vi "getSquareCoordinates.vi"(10 "Grid":T2, 11 "square":T1) -> (3 "Cluster":cluster{dbl, dbl, dbl, dbl})   [LabVIEW 2020]
uses:
  <vilib>/imath/engines/lvmath2/RunTimeEngine/NodeEndStatement/NIMS_NodeEndStatement_Output.vi
  <instcachedir>/0/NIMS_NodeEndStatement_Output_53EC0D466D134D7ABD903AC30B43404B.lvgen/NIMS_NodeEndStatement_Output_53EC0D466D134D7ABD903AC30B43404B_000.vi
  <vilib>/imath/engines/lvmath2/RunTimeEngine/ErrorHandling/NIMS_Finalize Error.vi
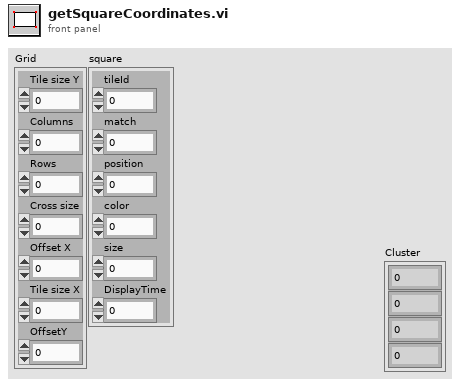
[diagram p1: front panel]
types:
  T1 = cluster{"tileId":i32, "match":i32, "position":i32, "color":u32, "size":i32, "DisplayTime":i32}
  T2 = cluster{"Tile size Y":dbl, "Columns":dbl, "Rows":dbl, "Cross size":dbl, "Offset X":dbl, "Tile size X":dbl, "OffsetY":dbl}
  T3 = cluster{"left":dbl, "top":dbl, "right":dbl, "bottom":dbl}
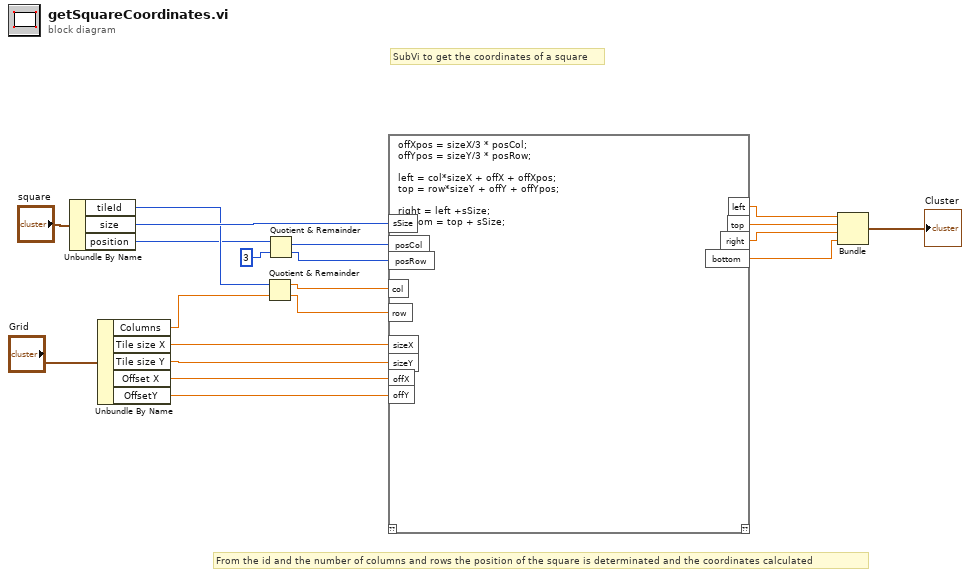
[diagram p0: block diagram]
diagram:
  # "From the id and the number of columns and rows the position of the square is determinated and the coordinates calculated"
  # "SubVi to get the coordinates of a square"
  n1 = Unbundle By Name("square") -> ("tileId"=w17:i32, "size"=w18:i32, "position"=w5:i32)
  n2 = Unbundle By Name("Grid") -> ("Columns"=w16:dbl, "Tile size X"=w13:dbl, "Tile size Y"=w12:dbl, "Offset X"=w11:dbl, "OffsetY"=w10:dbl)
  n3 = Quotient & Remainder(x=w17, y=w16) -> (x-y*floor(x/y)=w15:dbl, floor(x/y)=w14:dbl)
  n4 = Quotient & Remainder(x=w5, y=3) -> (x-y*floor(x/y)=w3:i32, floor(x/y)=w2:i32)
  n5 = mathscript code="offXpos = sizeX/3 * posCol;\noffYpos = sizeY/3 * posRow;\n\nleft = col*sizeX + offX + offXpos;\ntop = row*sizeY + offY + offYpos;\n\nright = left +sSize;\nbottom = top + sSize;"("col"=w15, "row"=w14, "sizeX"=w13, "sizeY"=w12, "sSize"=w18, "offX"=w11, "offY"=w10, "posCol"=w3, "posRow"=w2) -> ("left"=w9:dbl, "top"=w8:dbl, "right"=w7:dbl, "bottom"=w6:dbl)  [unwired: 1 in, 1 out]
  n6 = Bundle("left"=w9, "top"=w8, "right"=w7, "bottom"=w6) -> (→"Cluster":T3)  [unwired: 1 in]
